vi "Fenstertitel uebersetzen.vi"(7 "Index (Seite)":i32, 8 "error in (no error)":errorcluster caption="Fehler (Eingang, kein Fehler)", 9 "Sprache verwenden":bool, 10 "Sprachauswahl":u16, 11 "Dieses VI":refnum<vi>) -> (0 "error out":errorcluster caption="Fehler (Ausgang)", 1 "Dieses VI out":refnum<vi>, 2 "Sprachauswahl out":u16, 3 "Sprachliste":string[][](array[string]))   [LabVIEW 2020, in "Sprachverwaltung.lvlib"]
uses:
  Sprachverwaltung.lvlib
  FGV Aktion Tabelle zerlegen.ctl
  Seiten/System Einstellungen V2/Aktioen FGV System Konstanten.ctl
  Seiten/System Einstellungen V2/System Einstellungen V2.lvlib
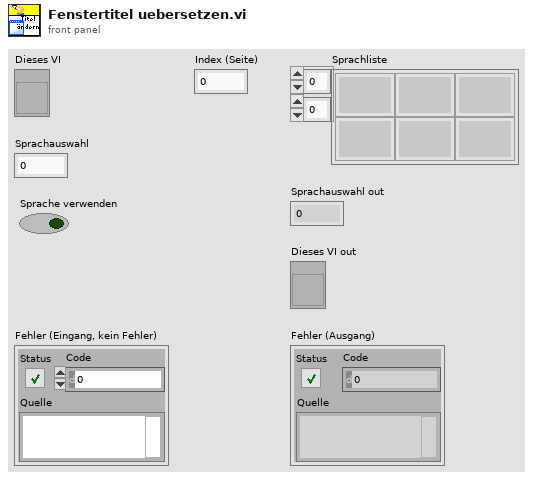
[diagram p1: front panel]
types:
  T1 = typedef "Sprachverwaltung.lvlib/FGV Aktion Tabelle zerlegen.ctl" = enum16{"laden", "vereinzeln", "speichern"}
  T2 = typedef "System Einstellungen V2.lvlib/Aktioen FGV System Konstanten.ctl" = enum16{"lesen", "laden", "speichern", "Sprache"}
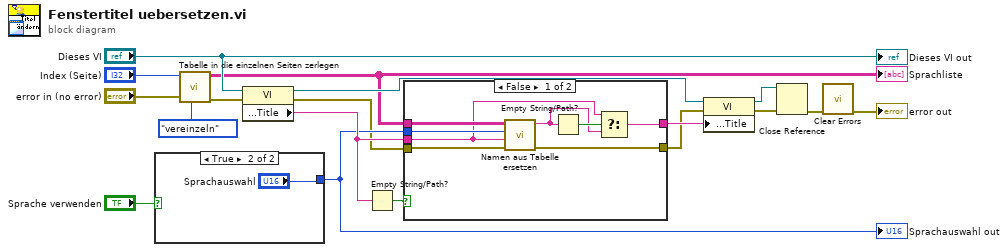
[diagram p0: block diagram]
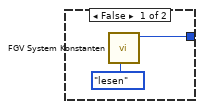
[diagram p2: hidden frame]
diagram:
  n1 = case shown="True" "Sprache verwenden" {
    tunnel: [w19 "Sprachauswahl"] -> w6
    frame False {
      n2 = call "FGV System Konstanten.vi"("Aktionen"=Aktioen_FGV_System_Konstanten."lesen") -> ("Sprachindex"=w19:u16)  [unwired: 6 in, 4 out]
    }
    frame True {
    }
  }
  "Sprachauswahl out" <- w6
  n3 = call "Tabelle in die einzelnen Seiten zerlegen.vi"("Aktion"=FGV_Aktion_Tabelle_zerlegen."vereinzeln", "error in (no error)"="error in (no error)", "Index (Seite)"="Index (Seite)") -> ("error out"=w4:errorcluster, "Sprachliste"=w12:string[][])  [unwired: 6 in, 1 out]
  "Sprachliste" <- w12
  n4 = property class="VI"(reference="Dieses VI", error in=w4) -> (reference out=w14:refnum<vi>, error out=w3:errorcluster, "Front Panel.Title"=w10:string)
  n5 = Empty String/Path?(string/path=w10) -> (empty?=w11:bool)
  n6 = case shown="False" w11 {
    tunnel: w12 -> [w29 _]
    tunnel: w6 -> [w28 _]
    tunnel: w10 -> [w26 w31]
    tunnel: [w24 w31] -> w9
    tunnel: w3 -> [w23 w30]
    tunnel: [w22 w30] -> w2
    frame False {
      n7 = call "Namen aus Tabelle ersetzen.vi"("Fehler (Eingang, kein Fehler)"=w23, "Regulärer Ausdruck"=w26, "Sprachauswahl"=w28, "Tabelle"=w29) -> ("Fehler (Ausgang)"=w22:errorcluster, "Übersetzung"=w25:string)  [unwired: 6 in]
      n8 = Empty String/Path?(string/path=w25) -> (empty?=w27:bool)
      n9 = Select(t=w26, s=w27, f=w25) -> (s? t:f=w24:string)
    }
    frame True {
    }
  }
  n10 = property class="VI"(reference=w14, error in=w2, "Front Panel.Title"=w9) -> (reference out=w16:refnum<vi>, error out=w17:errorcluster)
  n11 = Close Reference(reference=w16, error in (no error)=w17) -> (error out=w15:errorcluster)
  n12 = call <vilib>:"Clear Errors.vi"("error in (no error)"=w15) -> ("error out"=→"error out":errorcluster)  [unwired: 5 in, 1 out]
  "Dieses VI out" <- "Dieses VI"
